vi "Get Multi-Line Package Attribute Value.vi"(8 "error in (no error)":errorcluster, 10 "package attribute name":string, 11 "package attributes CLI string":string) -> (0 "error out":errorcluster, 2 "description":string, 3 "synopsis":string)   [LabVIEW 2014, in "NIPM_API.lvlib"]
uses:
  NIPM_API.lvlib
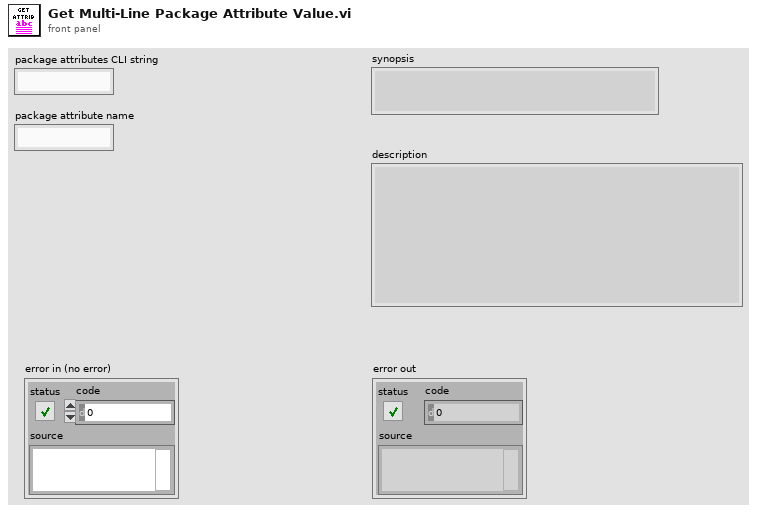
[diagram p1: front panel]
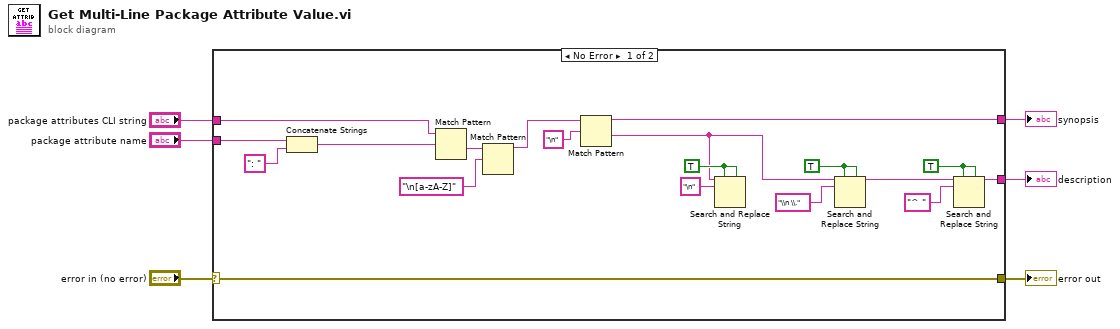
[diagram p0: block diagram]
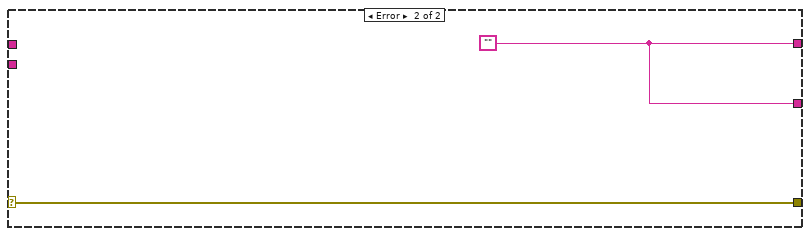
[diagram p2: hidden frame]
diagram:
  n1 = case shown="No Error" "error in (no error)" {
    selector: "error in (no error)" -> [w19 w27]
    tunnel: "package attributes CLI string" -> [w25 _]
    tunnel: "package attribute name" -> [w21 _]
    tunnel: [w15 w26] -> w5
    tunnel: [w19 w27] -> w3
    tunnel: [w8 w26] -> w2
    frame No Error {
      w10 = TRUE ("replace all? (F)")
      w13 = TRUE ("replace all? (F)")
      w14 = TRUE ("replace all? (F)")
      n2 = Concatenate Strings(w21, ": " ("regular expression")) -> (w20:string)
      n3 = Match Pattern(string=w25, regular expression=w20) -> (after substring=w24:string)  [unwired: 1 in, 3 out]
      n4 = Match Pattern(string=w24, regular expression="\n[a-zA-Z]" ("Package Attribute Name")) -> (before substring=w16:string)  [unwired: 1 in, 3 out]
      n5 = Match Pattern(string=w16, regular expression="\n") -> (before substring=w15:string, after substring=w11:string)  [unwired: 1 in, 2 out]
      n6 = Search and Replace String(replace all?=w13, multiline?=w13, input string=w11, search string="\n") -> ()  [unwired: 4 in, 4 out]
      n7 = Search and Replace String(replace all?=w14, multiline?=w14, input string=w11, search string="\\n \\.") -> (result string=w7:string)  [unwired: 4 in, 3 out]
      n8 = Search and Replace String(replace all?=w10, multiline?=w10, input string=w7, search string="^ ") -> (result string=w8:string)  [unwired: 4 in, 3 out]
    }
    frame Error {
      w26 = ""
    }
  }
  "synopsis" <- w5
  "error out" <- w3
  "description" <- w2
